vi "Get Count.vi"(8 "error in (no error)":errorcluster, 11 "Core Plugins Configuration in":refnum<class "Core Plugins Configuration.lvclass">) -> (0 "error out":errorcluster, 2 "count":i32, 3 "Core Plugins Configuration out":refnum<class "Core Plugins Configuration.lvclass">)   [LabVIEW 2017, in "DSF Core.lvlib" / "Core Plugins Configuration.lvclass"]
uses:
  Core Plugins Configuration.lvclass
  Core Plugins Configuration.lvclass/Core Plugins Configuration.ctl
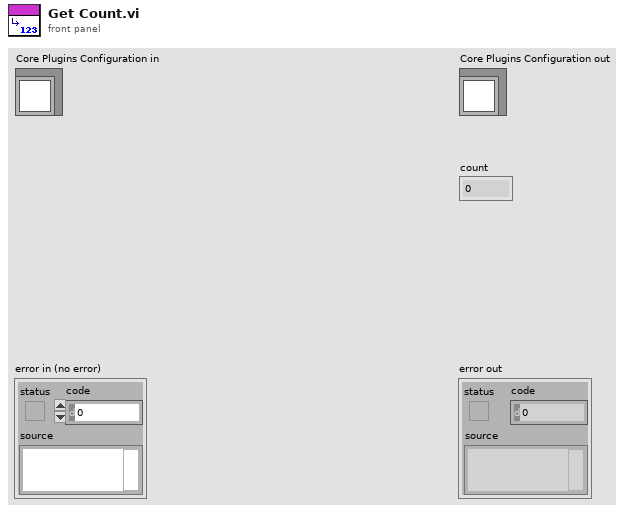
[diagram p1: front panel]
types:
  T1 = typedef "DSF Core.lvlib/Core Plugins Configuration.lvclass/Configuration.ctl" = cluster{"name":string, "components":string[], "cycle timing":T2}
  T2 = typedef "DSF Core.lvlib/DSF Timing Info.ctl" = cluster{"priority":u64, "decimation":u64, "offset":u64}
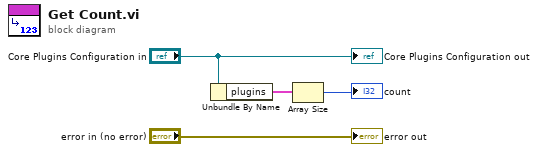
[diagram p0: block diagram]
diagram:
  n1 = Unbundle By Name("Core Plugins Configuration in") -> ("plugins"=w3:T1[])
  n2 = Array Size(array=w3) -> (size(s)=→"count":i32)
  "error out" <- "error in (no error)"
  "Core Plugins Configuration out" <- "Core Plugins Configuration in"
